vi "Wago notifier.vi"(6 "Operation":enum16{"Init", "Get", "Set"}(ring)=enum."Get", 8 "error in":errorcluster, 11 "notifier out 2":refnum<notifier>) -> (0 "error out":errorcluster, 3 "notifier out":refnum<notifier>)   [LabVIEW 2021]
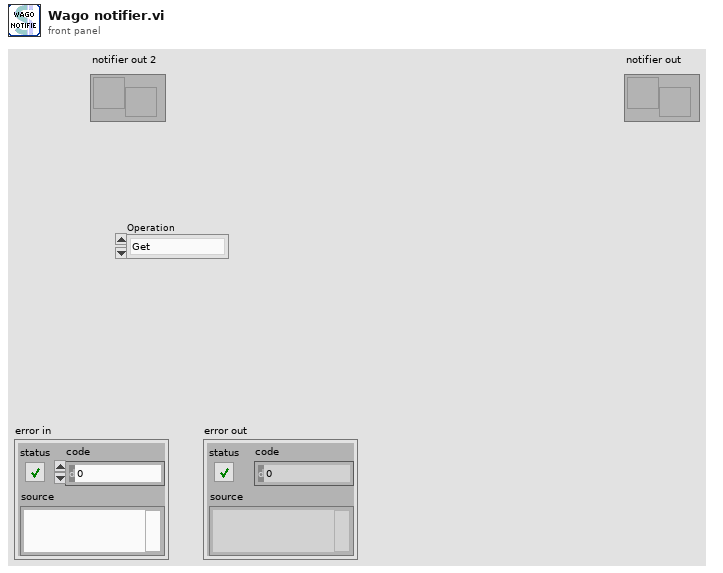
[diagram p1: front panel]
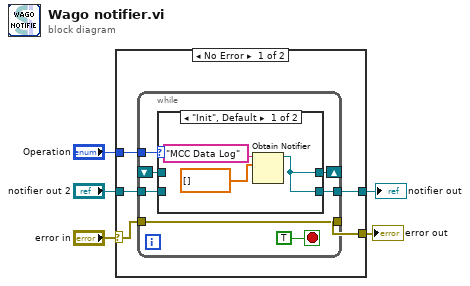
[diagram p0: block diagram]
diagram:
  n1 = case shown="No Error" "error in" {
    selector: "error in" -> [w8 w23]
    tunnel: "Operation" -> [w10 _]
    tunnel: [w9 w22] -> w2
    tunnel: [w7 w23] -> w3
    tunnel: "notifier out 2" -> [w6 w22]
    frame No Error {
      n2 = while {
        tunnel: w10 -> [w16]
        tunnel: w6 -> [w15]
        shift-right: [w14] -> _
        shift-left: _ -> [w12]
        tunnel: [w13] -> w9
        tunnel: w8 -> [w11]
        tunnel: [w11] -> w7
        stop <- TRUE stop-if-true
        n3 = case shown="\"Init\", Default" w16 {
          tunnel: w15 -> [_ _]
          tunnel: [w18 w21] -> w14
          tunnel: [w18 w21] -> w13
          tunnel: w12 -> [_ w21]
          frame "Init", Default {
            n4 = Obtain Notifier(name (unnamed)="MCC Data Log", notification data type=sgl[] [] ("initialized array")) -> (notifier out=w18:refnum<notifier>)  [unwired: 2 in, 2 out]
          }
          frame "Get" {
          }
        }
      }
    }
    frame Error {
    }
  }
  "error out" <- w3
  "notifier out" <- w2
